vi "Obtain Broadcast Events for Registration.vi"(8 "error in":errorcluster) -> (0 "error out":errorcluster, 2 "Already running?":bool, 3 "Display Data Broadcast Events":T1)   [LabVIEW 2020, in "Display Data.lvlib"]
doc: "Return the broadcast event refnums so the module's caller can register for the module's broadcast events.\n_____\nBased on DQMH Project Template 6.1.0.94."
uses:
  Display Data.lvlib
  Broadcast Events--cluster.ctl
  Did Init Argument--cluster.ctl
  Status Updated Argument--cluster.ctl
  Error Reported Argument--cluster.ctl
  Stop Argument--cluster.ctl
  Get Module Execution Status Argument--cluster.ctl
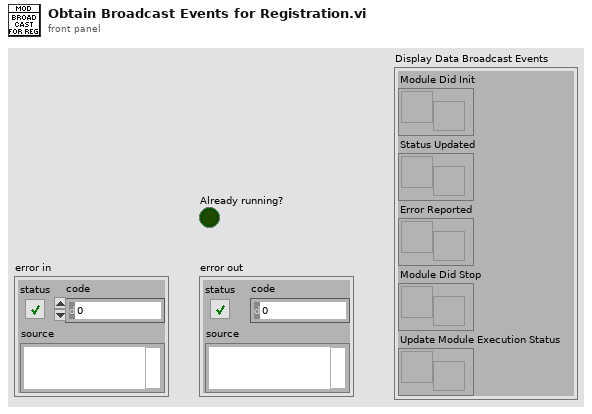
[diagram p1: front panel]
types:
  T1 = typedef "Display Data.lvlib/Broadcast Events--cluster.ctl" = cluster{"Module Did Init":refnum<user-event>, "Status Updated":refnum<user-event>, "Error Reported":refnum<user-event>, "Module Did Stop":refnum<user-event>, "Update Module Execution Status":refnum<user-event>}
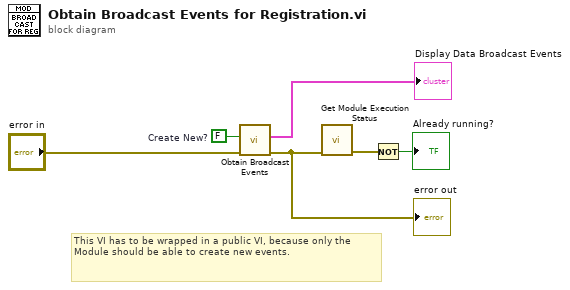
[diagram p0: block diagram]
diagram:
  w5 = FALSE  # Create New?
  # "This VI has to be wrapped in a public VI, because only the Module should be able to create new events."
  n1 = call "Obtain Broadcast Events.vi"("error in (no error)"="error in", "Create New? (F)"=w5) -> ("error out"=w3:errorcluster, "Display Data Broadcast Events"=→"Display Data Broadcast Events":T1)  [unwired: 8 in]
  "error out" <- w3
  n2 = call "Get Module Execution Status.vi"("error in (no error)"=w3) -> ("error out"=w2:errorcluster)  [unwired: 10 in]
  n3 = Not(x=w2) -> (.not. x?=→"Already running?":bool)
